vi "Add Child.vi"(8 "error in (no error)":errorcluster, 10 "Child":i32, 11 "Config Element in":refnum<class "Config Element.lvclass">) -> (0 "error out":errorcluster, 3 "Config Element out":refnum<class "Config Element.lvclass">)   [LabVIEW 2020, in "CDM-Config.lvlib" / "Config Element.lvclass"]
uses:
  Config Element.lvclass
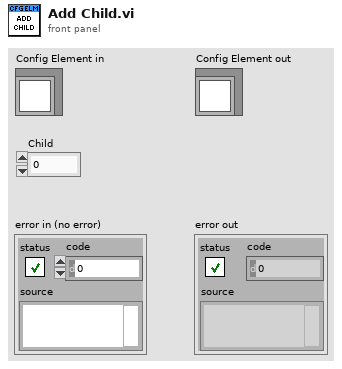
[diagram p1: front panel]
types:
  T1 = typedef "CDM-Config.lvlib/Config Element.lvclass/Ref Data.ctl" = cluster{"Node Info":T2, "Owner":refnum<class>, "Changed":bool, "Name":string, "Value":string, "Meta Data":T3[]}
  T2 = typedef "CDM-Config.lvlib/Node Info.ctl" = cluster{"Index":i32, "Parent":i32, "Children":i32[]}
  T3 = typedef "CDM-Config.lvlib/Meta Data.ctl" = cluster{"Name":string, "Value":string}
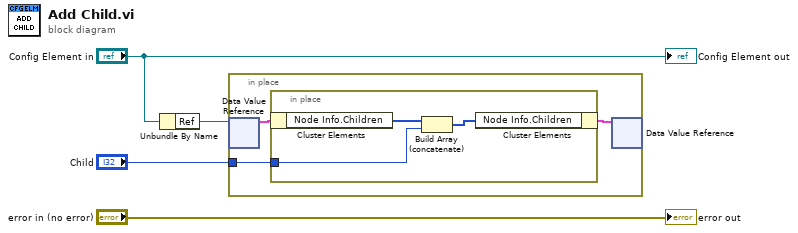
[diagram p0: block diagram]
diagram:
  n1 = Unbundle By Name("Config Element in") -> ("Ref"=w3:refnum<data-value>)
  n2 = in-place {
    in-place-border: "Child" -> [w5]
    n3 = in-place-dvr #1(w3) -> (w7:T1)  [unwired: 1 out]
    n4 = in-place {
      in-place-border: w5 -> [w9]
      n5 = in-place-cluster #2(w7) -> ("Node Info.Children"=w10:i32[])
      n6 = Build Array (concatenate)(w10, w9) -> (w8:i32[])
      n7 = in-place-cluster #2("Node Info.Children"=w8) -> (w6:T1)
    }
    n8 = in-place-dvr #1(w6) -> ()  [unwired: 2 out]
  }
  "error out" <- "error in (no error)"
  "Config Element out" <- "Config Element in"
